vi "Get Hardware Configuration File.vi"(8 "error in":errorcluster, 11 "Ballard MIL-STD 1553 custom device in":T1 format="%.0x") -> (0 "error out":errorcluster, 1 "RT destination":path, 2 "hardware configuration file":path, 3 "Ballard MIL_STD 1553 custom device out":T1 format="%.0x")   [LabVIEW 2020, in "AIM MIL-STD-1553 Scripting.lvlib"]
doc: "Returns the <b>hardware configuration file</b>. The hardware configuration file must be consistent with system configuration for successful deployment and avionics bus communication."
uses:
  AIM MIL-STD-1553 Scripting.lvlib
  <vilib>/NI VeriStand/Custom Device API/Custom Device Item Ref.ctl
  Constants.vi
  <vilib>/NI VeriStand/Custom Device API/Get Item Property (Dependent File).vi
  <vilib>/NI VeriStand/Custom Device API/Custom Device API.lvlib
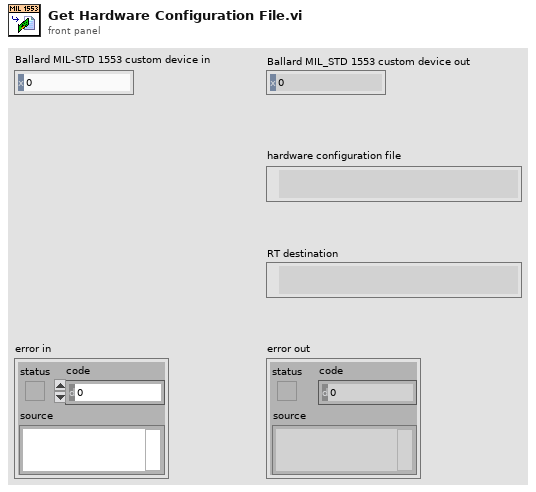
[diagram p1: front panel]
types:
  T1 = typedef "Custom Device API.lvlib/Custom Device Item Ref.ctl" = u64
  T2 = typedef "Custom Device API.lvlib/Dependent File Optional Info.ctl" = cluster{"Version":string, "RTDestination":path, "ForceDownload":bool, "SupportedTarget":string, "MD5":string}
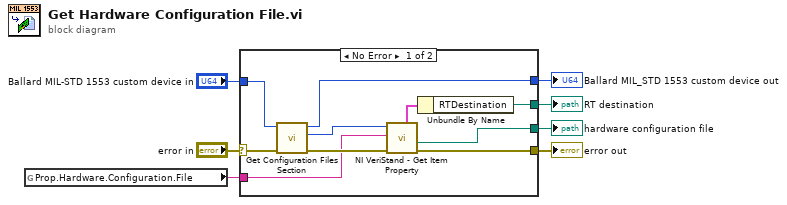
[diagram p0: block diagram]
diagram:
  n1 = global read "Constants.vi" "Prop.Hardware.Configuration.File"() -> (w1:string)
  n2 = case shown="No Error" "error in" {
    selector: "error in" -> [w13 w19]
    tunnel: "Ballard MIL-STD 1553 custom device in" -> [w16 w18]
    tunnel: [w14 w18] -> w6
    tunnel: [w11 w19] -> w4
    tunnel: [w10 _] -> w3
    tunnel: [w9 _] -> w2
    tunnel: w1 -> [w8 _]
    frame No Error {
      n3 = call "Get Configuration Files Section.vi"("error in"=w13, "custom device in"=w16) -> ("error out"=w12:errorcluster, "configuration files section"=w15:T1, "custom device out"=w14:T1)  [unwired: 6 in, 1 out]
      n4 = call-poly <vilib>:"NI VeriStand - Get Item Property.vi"("error in (no error)"=w12, "Property Name"=w8, "Item Ref in"=w15) -> ("error out"=w11:errorcluster, "Path"=w9:path, "OptionalInfo"=w17:T2)  [unwired: 4 in, 2 out]
      n5 = Unbundle By Name(w17) -> ("RTDestination"=w10:path)
    }
    frame Error {
    }
  }
  "error out" <- w4
  "hardware configuration file" <- w2
  "Ballard MIL_STD 1553 custom device out" <- w6
  "RT destination" <- w3
